vi "Driver Validate File.vi"(4 "Drivers Folder (Empty)":path, 5 "error in (no error)":errorcluster, 6 "Driver Filename Extension (\"\")":string, 7 "sType(\"\")":string, 8 "sxDriverId (\"\")":string) -> (0 "error out":errorcluster, 1 "Valid?":bool, 3 "Driver Record":T1)   [LabVIEW 2011]
uses:
  Driver Record.ctl
  Summitek EXT/Miscellaneous/OGAB Version.ctl
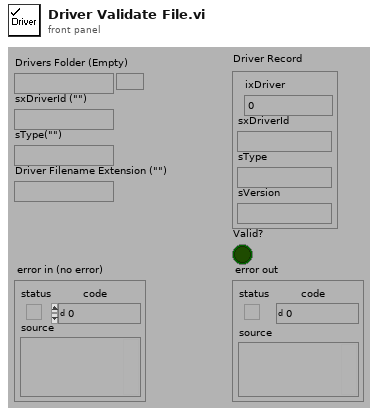
[diagram p1: front panel]
types:
  T1 = typedef "Driver Record.ctl" = cluster{"ixDriver":i32, "sxDriverId":string, "sType":string, "sVersion":string}
  T2 = enum32{"invalid app kind", "Development System", "Run Time System", "Student Edition", "Embedded LabVIEW", "Evaluation", "Custom"}
  T3 = typedef "OGAB Version.ctl" = cluster{"Version":string, "Build Number":u32, "Build Date/Time":dbl}
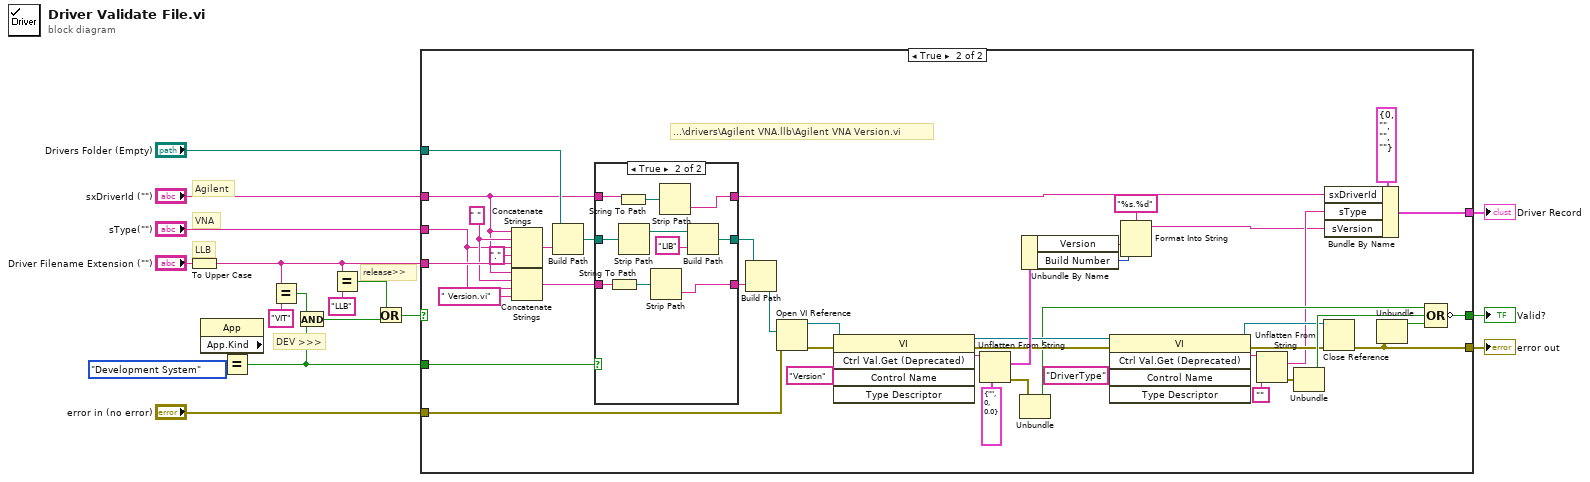
[diagram p0: block diagram]
diagram:
  # "LLB"
  # "DEV >>>"
  # "release>>"
  # "VNA"
  # "Agilent"
  n1 = To Upper Case(1:"Driver Filename Extension (\"\")") -> (0:w7:string)
  n2 = property class="App"() -> ("App.Kind"=w9:T2)  [unwired: 2 in, 2 out]
  n3 = Equal?(x=w9, y=T2."Development System") -> (x = y?=w2:bool)
  n4 = Equal?(x=w7, y="VIT") -> (x = y?=w5:bool)
  n5 = And(x=w5, y=w2) -> (x .and. y?=w4:bool)
  n6 = Equal?(x=w7, y="LLB") -> (x = y?=w6:bool)
  n7 = Or(x=w6, y=w4) -> (x .or. y?=w3:bool)
  n8 = case shown="True" w3 {
    selector: w3 -> [w19 _]
    tunnel: "error in (no error)" -> [w20 w63]
    tunnel: "Drivers Folder (Empty)" -> [_ w61]
    tunnel: "sxDriverId (\"\")" -> [_ w29]
    tunnel: [w19 w47] -> w13
    tunnel: [w20 w49] -> w12
    tunnel: w7 -> [_ w40]
    tunnel: "sType(\"\")" -> [_ w38]
    tunnel: w2 -> [_ w21]
    tunnel: [_ w23] -> w1
    frame False {
    }
    frame True {
      w39 = " "
      # "...\\drivers\\Agilent VNA.llb\\Agilent VNA Version.vi"
      n9 = Concatenate Strings(w29, w39, w38, ".", w40) -> (w60:string)
      n10 = Concatenate Strings(w29, w39, w38, " Version.vi") -> (w31:string)
      n11 = Build Path(base path=w61, name or relative path=w60) -> (appended path=w33:path)
      n12 = case shown="True" w21 {
        tunnel: [w66 w71] -> w32
        tunnel: w33 -> [w66 w73]
        tunnel: w31 -> [w65 w76]
        tunnel: [w65 w74] -> w30
        tunnel: w29 -> [w64 w68]
        tunnel: [w64 w67] -> w28
        frame False {
        }
        frame True {
          n13 = String To Path(string=w76) -> (path=w75:path)
          n14 = String To Path(string=w68) -> (path=w69:path)
          n15 = Strip Path(path=w73) -> (stripped path=w72:path)  [unwired: 1 out]
          n16 = Strip Path(path=w75) -> (name=w74:string)  [unwired: 1 out]
          n17 = Strip Path(path=w69) -> (name=w67:string)  [unwired: 1 out]
          n18 = Build Path(base path=w72, name or relative path="LIB") -> (appended path=w71:path)
        }
      }
      n19 = Build Path(base path=w32, name or relative path=w30) -> (appended path=w34:path)
      n20 = Open VI Reference(vi path=w34, error in (no error)=w63) -> (vi reference=w58:refnum<vi>, error out=w59:errorcluster)  [unwired: 4 out]
      n21 = invoke class="VI" method="Ctrl Val.Get (Deprecated)"(reference=w58, error in=w59, "Control Name"="Version") -> (reference out=w50:refnum<vi>, error out=w51:errorcluster, "Get Control Value"=w56:string)  [unwired: 2 in, 2 out]
      n22 = Unflatten From String(type=T3 {"Version"="", "Build Number"=0, "Build Date/Time"=0.0} ("Version"), binary string=w56) -> (value=w54:T3, error out=w35:errorcluster)  [unwired: 1 in, 3 out]
      n23 = Unbundle(w35) -> ("status"=w45:bool)  [unwired: 2 out]
      n24 = Unbundle By Name(w54) -> ("Version"=w26:string, "Build Number"=w25:u32)
      n25 = invoke class="VI" method="Ctrl Val.Get (Deprecated)"(reference=w50, error in=w51, "Control Name"="DriverType") -> (reference out=w43:refnum<vi>, error out=w42:errorcluster, "Get Control Value"=w53:string)  [unwired: 2 in, 2 out]
      n26 = Format Into String(format string="%s.%d", w26, w25) -> (resulting string=w24:string)  [unwired: 2 in, 1 out]
      n27 = Unflatten From String(type="", binary string=w53) -> (value=w41:string, error out=w36:errorcluster)  [unwired: 1 in, 3 out]
      n28 = Unbundle(w36) -> ("status"=w46:bool)  [unwired: 2 out]
      n29 = Close Reference(reference=w43, error in (no error)=w42) -> (error out=w49:errorcluster)
      n30 = Bundle By Name(cluster=T1 {"ixDriver"=0, "sxDriverId"="", "sType"="", "sVersion"=""} ("Driver Record"), "sxDriverId"=w28, "sType"=w41, "sVersion"=w24) -> (w23:T1)
      n31 = Unbundle(w49) -> ("status"=w48:bool)  [unwired: 2 out]
      n32 = Compound Arithmetic op=OR(w45, w46, w48) -> (invert w47:bool)
    }
  }
  "error out" <- w12
  "Valid?" <- w13
  "Driver Record" <- w1
